vi "DAC Configure.vi"(8 "error in":errorcluster, 11 "DAC Keller PAA25 in":refnum<class "DAC Keller PAA25.lvclass">) -> (0 "error out":errorcluster, 3 "DAC Keller PAA25 out":refnum<class "DAC Keller PAA25.lvclass">)   [LabVIEW 2019, in "DAC.lvlib" / "DAC Keller PAA25.lvclass"]
uses:
  DAC Keller PAA25.lvclass
  C:/Users/krio/Documents/LV_Projects/test-stand/App/DAC/DAC.lvclass
  DAC.lvclass/DAC.ctl
  DAC Keller PAA25.lvclass/DAC Keller PAA25.ctl
  <vilib>/DAQmx/create/channels.llb/DAQmx Create Channel (AI-Voltage-Basic).vi
  DAC.lvclass
  <vilib>/DAQmx/configure/timing.llb/DAQmx Timing (Sample Clock).vi
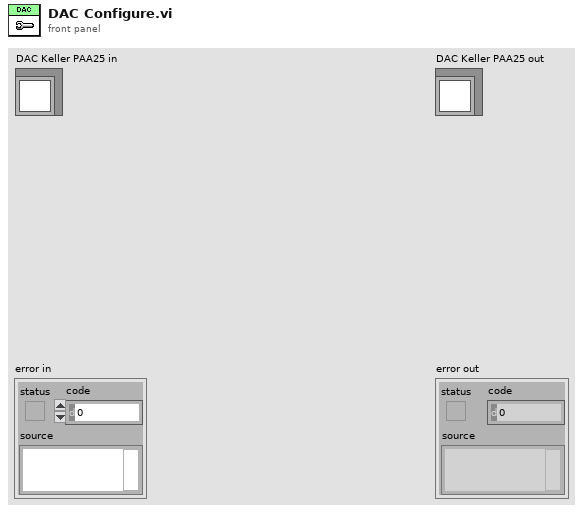
[diagram p1: front panel]
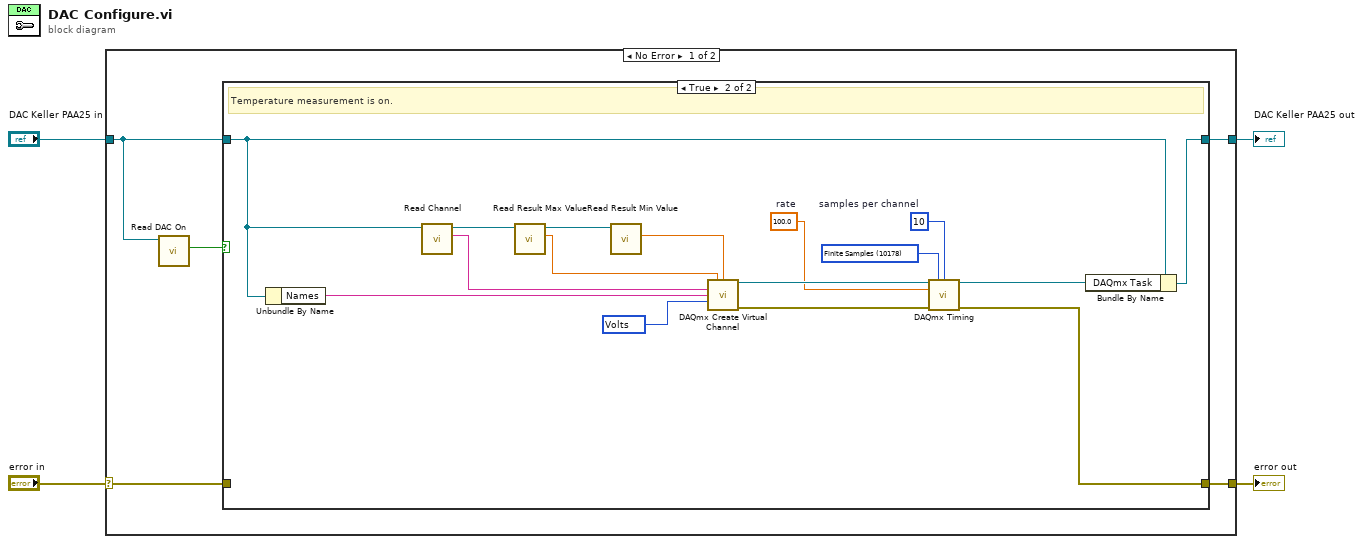
[diagram p0: block diagram]
diagram:
  n1 = case shown="No Error" "error in" {
    selector: "error in" -> [w6 w29]
    tunnel: [w5 w29] -> w4
    tunnel: [w7 w28] -> w3
    tunnel: "DAC Keller PAA25 in" -> [w9 w28]
    frame No Error {
      n2 = call "Read DAC On.vi"("DAC in"=w9) -> ("DAC On"=w8:bool)  [unwired: 8 in, 2 out]
      n3 = case shown="True" w8 {
        tunnel: w9 -> [w11 w25]
        tunnel: [w11 w27] -> w7
        tunnel: w6 -> [w10 _]
        tunnel: [w10 w15] -> w5
        frame False {
          # "Temperature measurement is off."
        }
        frame True {
          w12 = 10  # samples per channel
          w13 = 100.0  # rate
          w14 = 10178 items=["Finite Samples"=10178, "Continuous Samples"=10123, "Hardware Timed Single Point"=12522] ("sample mode")
          w19 = 10348 items=["Volts"=10348, "From Custom Scale"=10065] ("units")
          # "Temperature measurement is on."
          n4 = Unbundle By Name(w25) -> ("Names"=w26:string)
          n5 = call "Read Channel.vi"("DAC in"=w25) -> ("Channel"=w24:string, "DAC out"=w23:refnum<class "DAC Keller PAA25.lvclass">)  [unwired: 8 in, 1 out]
          n6 = call "Read Result Max Value.vi"("DAC in"=w23) -> ("Max Value"=w20:dbl, "DAC out"=w22:refnum<class "DAC Keller PAA25.lvclass">)  [unwired: 8 in, 1 out]
          n7 = call "Read Result Min Value.vi"("DAC in"=w22) -> ("Min Value"=w21:dbl)  [unwired: 8 in, 2 out]
          n8 = call-poly <vilib>:"DAQmx Create Virtual Channel.vi"("maximum value"=w20, "minimum value"=w21, "physical channels"=w24, "name to assign"=w26, "units"=w19) -> ("task out"=w18:refnum<k21>, "error out"=w17:errorcluster)  [unwired: 9 in]
          n9 = call-poly <vilib>:"DAQmx Timing.vi"("task/channels in"=w18, "sample mode"=w14, "samples per channel"=w12, "rate"=w13, "error in"=w17) -> ("task out"=w16:refnum<k21>, "error out"=w15:errorcluster)  [unwired: 9 in]
          n10 = Bundle By Name(cluster=w25, "DAQmx Task"=w16) -> (w27:refnum<class "DAC Keller PAA25.lvclass">)
        }
      }
    }
    frame Error {
    }
  }
  "error out" <- w4
  "DAC Keller PAA25 out" <- w3
